vi "Pumpentest.vi"() -> ()   [LabVIEW 2024]
uses:
  Treiber/Motor Treiber/Motor Treiber.lvlib
panel:
  in  "Start":bool
  in  "Angestrebte Max. Drehzahl":dbl
  in  "Abbauzeit":dbl
  in  "Haltezeit":u32
  in  "Aufbauzeit":dbl
  in  "stop":bool
  in  "Drehzahl Soll":dbl
  out "Drehzahl Ist":dbl
  out "Volumenstrom":dbl
  out "Druck":dbl
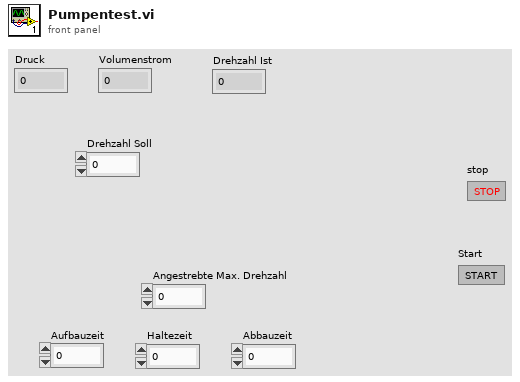
[diagram p1: front panel]
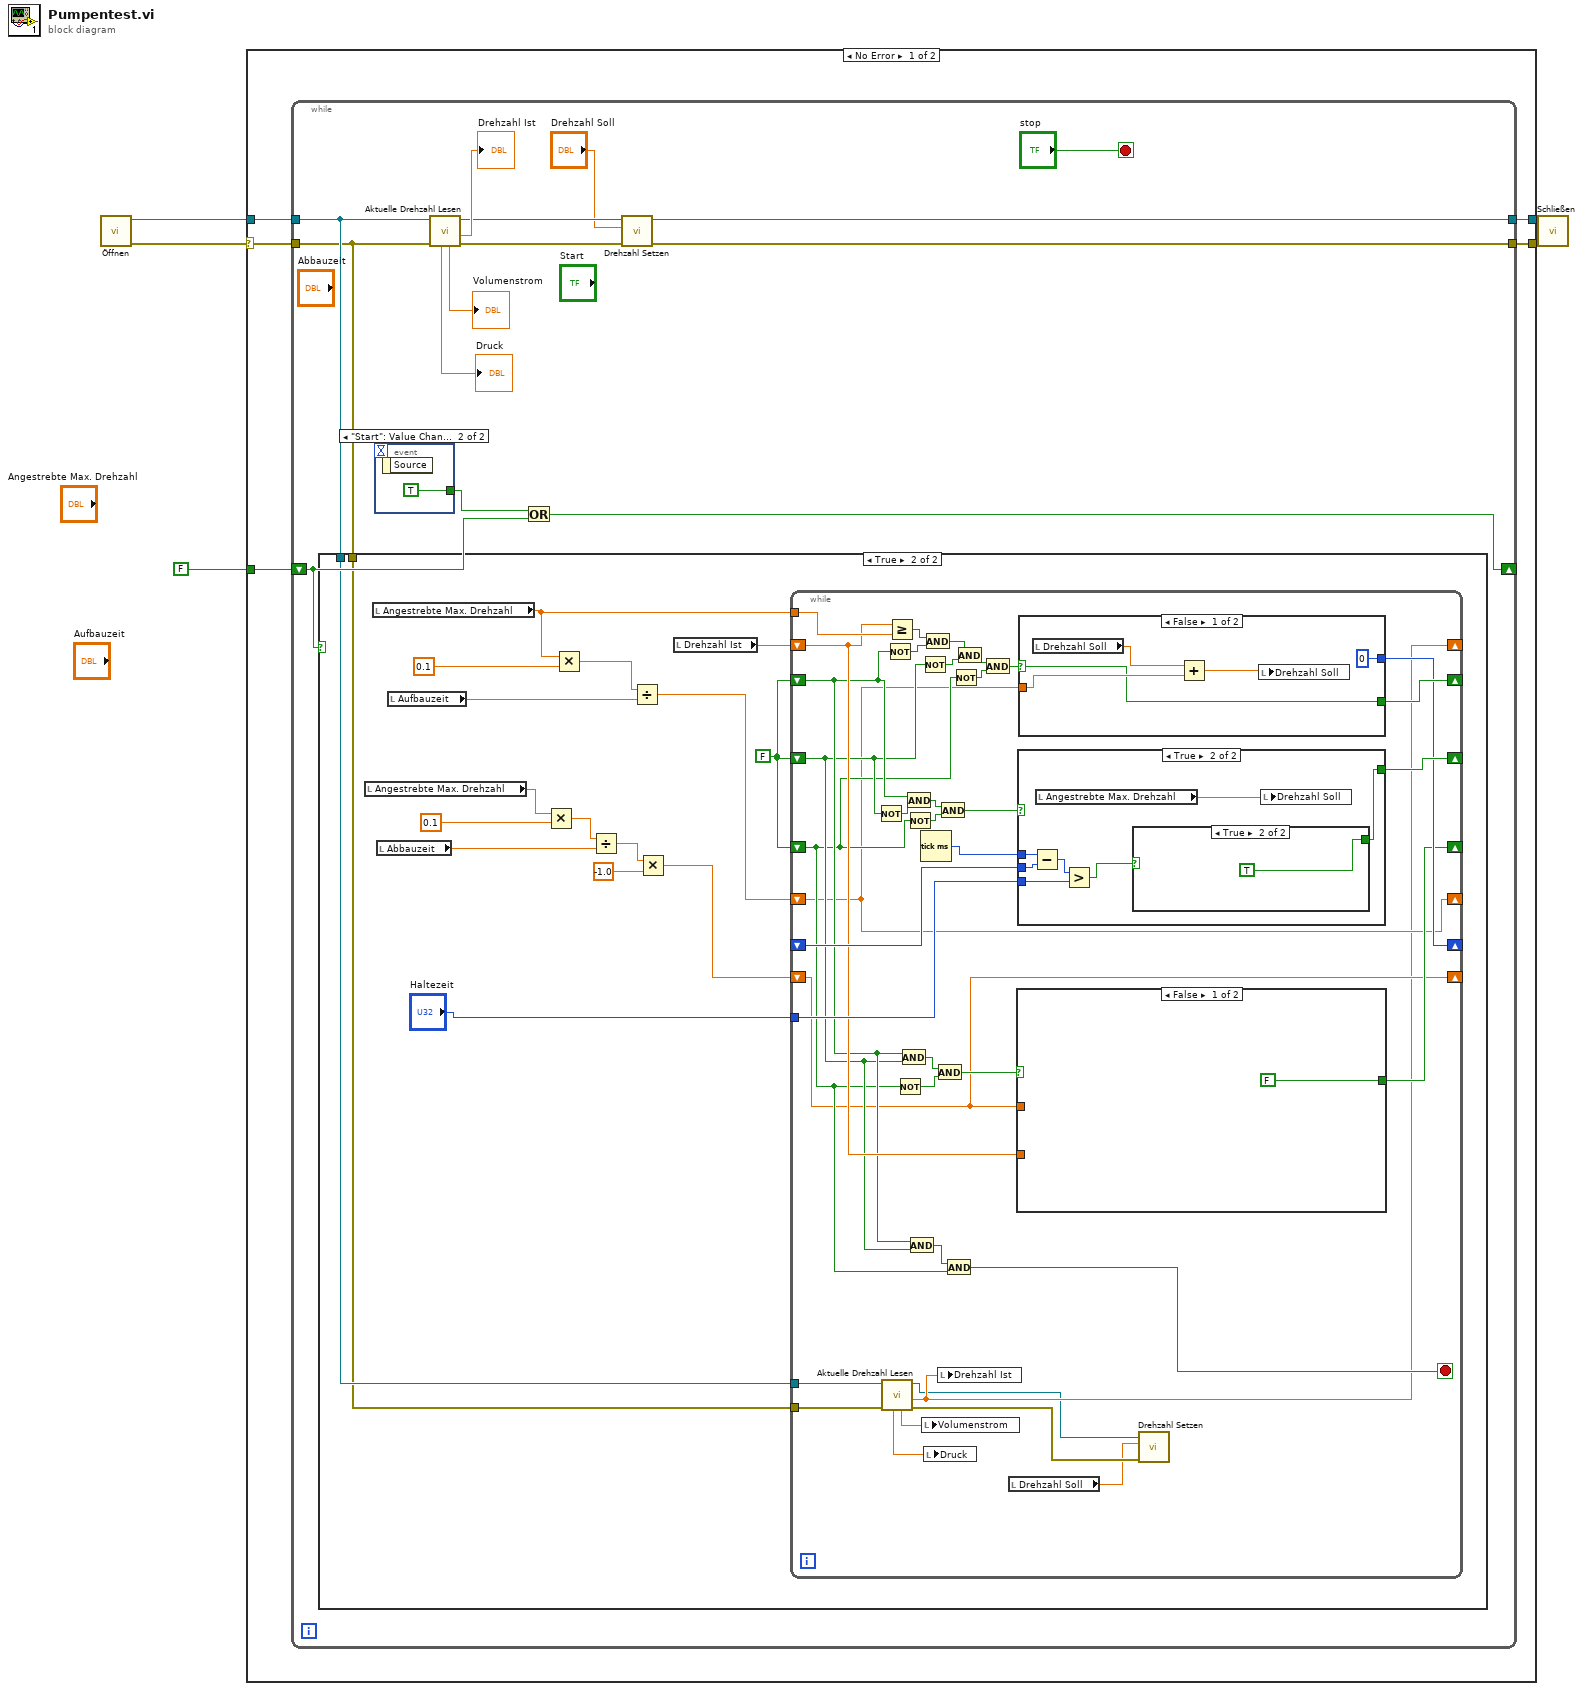
[diagram p0: block diagram]
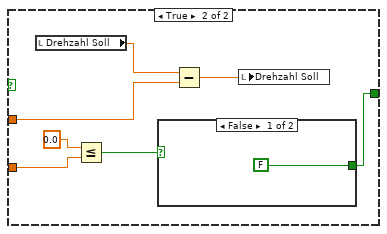
[diagram p3: hidden frame]
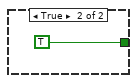
[diagram p4: hidden frame]
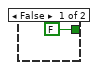
[diagram p5: hidden frame]
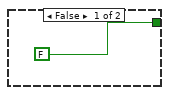
[diagram p6: hidden frame]
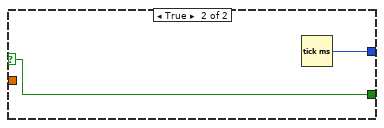
[diagram p7: hidden frame]
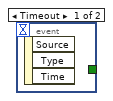
[diagram p8: hidden frame]
diagram:
  n1 = call "Öffnen.vi"() -> ("Error Out"=w5:errorcluster, "connection ID"=w4:refnum<k5>)  [unwired: 10 in]
  n2 = case shown="No Error" w5 {
    selector: w5 -> [w9 w108]
    tunnel: w4 -> [w10 w109]
    tunnel: [w8 w109] -> w3
    tunnel: [w7 w108] -> w2
    tunnel: FALSE -> [w6 _]
    frame No Error {
      n3 = while {
        tunnel: w10 -> [w13]
        tunnel: w9 -> [w12]
        tunnel: [w18] -> w8
        tunnel: [w11] -> w7
        shift-right: [w15] -> _
        shift-left: w6 -> [w14]
        stop <- "stop" stop-if-true
        n4 = case shown="True" w14 {
          tunnel: w13 -> [_ w26]
          tunnel: w12 -> [_ w25]
          frame False {
          }
          frame True {
            w41 = FALSE
            n5 = local read "Angestrebte Max. Drehzahl"() -> (w35:dbl)
            n6 = local read "Angestrebte Max. Drehzahl"() -> (w29:dbl)
            n7 = local read "Abbauzeit"() -> (w33:dbl)
            n8 = local read "Aufbauzeit"() -> (w38:dbl)
            n9 = Multiply(x=w35, y=0.1) -> (x*y=w34:dbl)
            n10 = Multiply(x=w29, y=0.1) -> (x*y=w39:dbl)
            n11 = Divide(x=w34, y=w33) -> (x/y=w32:dbl)
            n12 = Divide(x=w39, y=w38) -> (x/y=w37:dbl)
            n13 = Multiply(x=w32, y=-1.0) -> (x*y=w30:dbl)
            n14 = local read "Drehzahl Ist"() -> (w28:dbl)
            n15 = while {
              shift-right: [w78] -> _
              shift-left: w41 -> [w56]
              shift-right: [w77] -> _
              shift-left: w41 -> [w55]
              shift-right: [w58] -> _
              shift-left: w41 -> [w53]
              shift-right: [w51] -> _
              shift-left: w37 -> [w51]
              shift-right: [w50] -> _
              shift-left: w30 -> [w50]
              tunnel: w29 -> [w79]
              shift-right: [w46] -> _
              shift-left: w28 -> [w57]
              shift-right: [w76] -> _
              shift-left: _ -> [w75]
              tunnel: "Haltezeit" -> [w73]
              tunnel: w26 -> [w49]
              tunnel: w25 -> [w48]
              stop <- w52 stop-if-true
              n16 = Not(x=w55) -> (.not. x?=w65:bool)
              n17 = call "Aktuelle Drehzahl Lesen.vi"("Error In"=w48, "connection_ID_In"=w49) -> ("Error Out"=w44:errorcluster, "Drehzahl U/Min"=w46:dbl, "connection_ID_Out"=w43:refnum<k5>, "Volumenstrom"=w47:dbl, "Druck"=w45:dbl)  [unwired: 3 in, 2 out]
              n18 = Not(x=w56) -> (.not. x?=w71:bool)
              n19 = Greater Or Equal?(x=w57, y=w79) -> (x >= y?=w72:bool)
              n20 = Not(x=w53) -> (.not. x?=w60:bool)
              n21 = And(x=w56, y=w55) -> (x .and. y?=w61:bool)
              n22 = And(x=w56, y=w65) -> (x .and. y?=w64:bool)
              n23 = Not(x=w53) -> (.not. x?=w63:bool)
              n24 = And(x=w56, y=w55) -> (x .and. y?=w54:bool)
              n25 = Not(x=w55) -> (.not. x?=w69:bool)
              n26 = Tick Count (ms)() -> (millisecond timer value=w74:u32)
              n27 = local write "Volumenstrom"(w47) -> ()
              n28 = And(x=w72, y=w71) -> (x .and. y?=w70:bool)
              n29 = local write "Druck"(w45) -> ()
              n30 = And(x=w61, y=w60) -> (x .and. y?=w59:bool)
              n31 = And(x=w64, y=w63) -> (x .and. y?=w62:bool)
              n32 = local write "Drehzahl Ist"(w46) -> ()
              n33 = And(x=w54, y=w53) -> (x .and. y?=w52:bool)
              n34 = Not(x=w53) -> (.not. x?=w66:bool)
              n35 = And(x=w70, y=w69) -> (x .and. y?=w68:bool)
              n36 = And(x=w68, y=w66) -> (x .and. y?=w67:bool)
              n37 = local read "Drehzahl Soll"() -> (w42:dbl)
              n38 = case shown="False" w59 {
                tunnel: [FALSE w81] -> w58
                tunnel: w50 -> [_ w86]
                tunnel: w57 -> [_ w83]
                frame False {
                }
                frame True {
                  n39 = local read "Drehzahl Soll"() -> (w87:dbl)
                  n40 = Less Or Equal?(x=0.0, y=w83) -> (x <= y?=w82:bool)
                  n41 = case shown="False" w82 {
                    tunnel: [FALSE TRUE] -> w81
                    frame False {
                    }
                    frame True {
                    }
                  }
                  n42 = Subtract(x=w87, y=w86) -> (x-y=w85:dbl)
                  n43 = local write "Drehzahl Soll"(w85) -> ()
                }
              }
              n44 = case shown="True" w62 {
                tunnel: [FALSE w91] -> w77
                tunnel: w75 -> [_ w96]
                tunnel: w74 -> [_ w95]
                tunnel: w73 -> [_ w93]
                frame False {
                }
                frame True {
                  n45 = Subtract(x=w95, y=w96) -> (x-y=w94:u32)
                  n46 = local read "Angestrebte Max. Drehzahl"() -> (w97:dbl)
                  n47 = Greater?(x=w94, y=w93) -> (0:w92:bool)
                  n48 = case shown="True" w92 {
                    tunnel: [FALSE TRUE] -> w91
                    frame False {
                    }
                    frame True {
                    }
                  }
                  n49 = local write "Drehzahl Soll"(w97) -> ()
                }
              }
              n50 = case shown="False" w67 {
                selector: w67 -> [w101 w106]
                tunnel: w51 -> [w104 _]
                tunnel: [w101 w106] -> w78
                tunnel: [u32 0 ("millisecond timer value") w105] -> w76
                frame False {
                  n51 = local read "Drehzahl Soll"() -> (w103:dbl)
                  n52 = Add(x=w103, y=w104) -> (x+y=w102:dbl)
                  n53 = local write "Drehzahl Soll"(w102) -> ()
                }
                frame True {
                  n54 = Tick Count (ms)() -> (millisecond timer value=w105:u32)
                }
              }
              n55 = call "Drehzahl Setzen.vi"("Error In"=w44, "Drehzahl U/Min"=w42, "connection_ID_In"=w43) -> ()  [unwired: 7 in, 2 out]
            }
          }
        }
        n56 = event shown="[1] \"Start\": Value Change" {
          selector: _ -> [_ _]
          dyn-events: _ -> [_ _]
          timeout: _ -> [_ _]
          tunnel: [_ TRUE] -> w16
          event Timeout {
            n57 = event-data() -> ()  [unwired: 1 in, 3 out]
          }
          event "Start": Value Change {
            n58 = event-data() -> ()  [unwired: 1 in, 1 out]
          }
        }
        n59 = call "Aktuelle Drehzahl Lesen.vi"("Error In"=w12, "connection_ID_In"=w13) -> ("Error Out"=w19:errorcluster, "Drehzahl U/Min"=→"Drehzahl Ist":dbl, "connection_ID_Out"=w21:refnum<k5>, "Volumenstrom"=→"Volumenstrom":dbl, "Druck"=→"Druck":dbl)  [unwired: 3 in, 2 out]
        n60 = Or(x=w16, y=w14) -> (x .or. y?=w15:bool)
        n61 = call "Drehzahl Setzen.vi"("Error In"=w19, "Drehzahl U/Min"="Drehzahl Soll", "connection_ID_In"=w21) -> ("Error Out"=w11:errorcluster, "connection_ID_Out"=w18:refnum<k5>)  [unwired: 7 in]
      }
    }
    frame Error {
    }
  }
  n62 = call "Schließen.vi"("Error In"=w2, "connection_ID_In"=w3) -> ()  [unwired: 9 in, 1 out]
